vi "Fault Handling.vi"(8 "error in (no error)":errorcluster, 10 "FaultCode":i32, 11 "OPC UA in":refnum<class "OPC UA.lvclass">) -> (0 "error out":errorcluster, 2 "Fault codes":cluster{"Bit":string, "Description":string}[](array[cluster]), 3 "OPC UA out":refnum<class "OPC UA.lvclass">)   [LabVIEW 2021, in "OPC UA.lvlib" / "OPC UA.lvclass"]
uses:
  OPC UA.lvclass
  OPC UA.lvclass/OPC UA.ctl
panel:
  out "Fault":bool
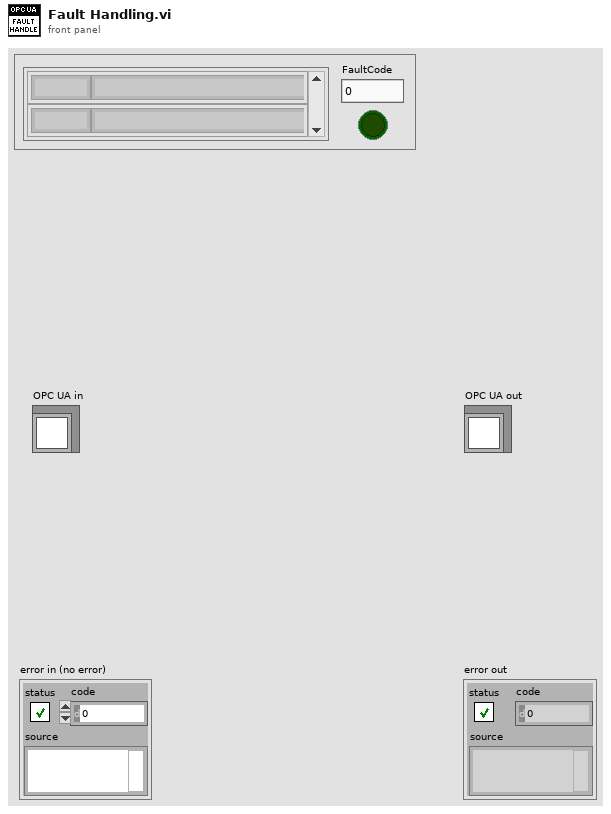
[diagram p1: front panel]
types:
  T1 = enum32{"Invalid", "Standard", "Closed", "Hidden", "Minimized", "Maximized"}
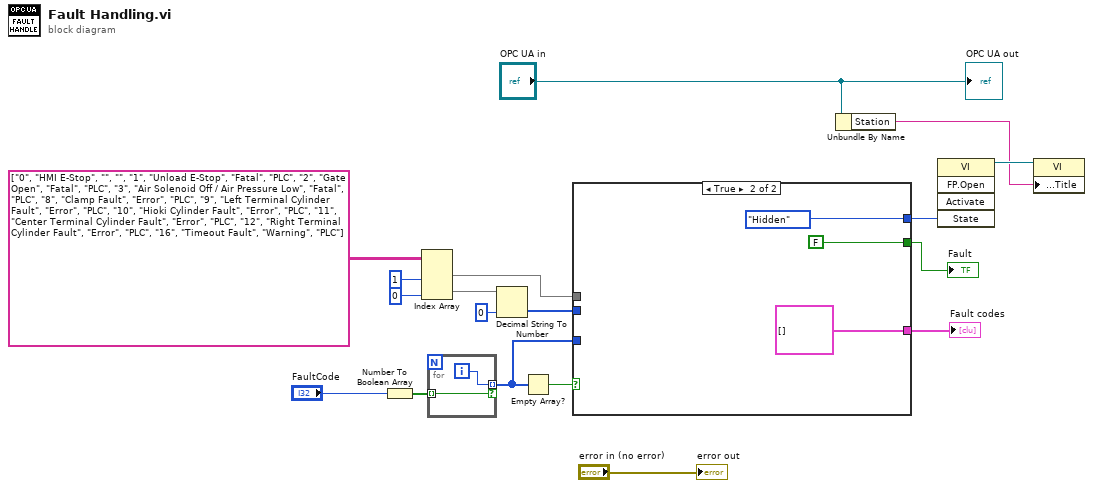
[diagram p0: block diagram]
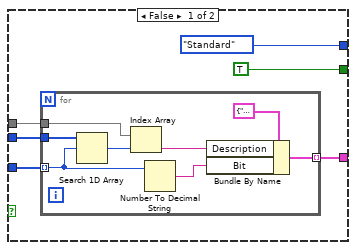
[diagram p2: hidden frame]
diagram:
  n1 = Number To Boolean Array(number="FaultCode") -> (Boolean array=w11:bool[])
  n2 = Index Array(array=string[][] [["0", "HMI E-Stop", "", ""], ["1", "Unload E-Stop", "Fatal", "PLC"], ["2", "Gate Open", "Fatal", "PLC"], ["3", "Air Solenoid Off / Air Pressure Low", "Fatal", "PLC"], ["8", "Clamp Fault", "Error", "PLC"], ["9", "Left Terminal Cylinder Fault", "Error", "PLC"], ["10", "Hioki Cylinder Fault", "Error", "PLC"], ["11", "Center Terminal Cylinder Fault", "Error", "PLC"], ["12", "Right Terminal Cylinder Fault", "Error", "PLC"], ["16", "Timeout Fault", "Warning", "PLC"]], index (col) #1=1 ("disabled index (col)"), index (col) #2=0 ("index (col)")) -> (element #1=w5:string[], element #2=w13:string[])  [unwired: 2 in]
  n3 = for {
    tunnel: w11 -> [w19] mode=indexing
    tunnel: [w20] -> w8 mode=indexing if=w19
    i -> [w20]
  }
  n4 = Decimal String To Number(string=w13, default (0L)=0 ("default (0 I32)")) -> (number=w7:i32[])  [unwired: 1 in, 1 out]
  n5 = Empty Array?(array=w8) -> (empty?=w6:bool)
  n6 = case shown="True" w6 {
    tunnel: [T1."Standard" ("State") T1."Hidden" ("State")] -> w14
    tunnel: [w21 cluster{"Bit":string, "Description":string}[] []] -> w2
    tunnel: [TRUE FALSE] -> w1
    tunnel: w7 -> [w24 _]
    tunnel: w8 -> [w23 _]
    tunnel: w5 -> [w22 _]
    frame False {
      n7 = for {
        tunnel: w23 -> [w29] mode=indexing
        tunnel: w24 -> [w34]
        tunnel: w22 -> [w32]
        tunnel: [w28] -> w21 mode=indexing
        n8 = Search 1D Array(1D array=w34, element=w29) -> (index of element=w33:i32)  [unwired: 1 in]
        n9 = Index Array(array=w32, index=w33) -> (element=w30:string)
        n10 = Number To Decimal String(number=w29) -> (decimal integer string=w27:string)  [unwired: 1 in]
        n11 = Bundle By Name(cluster=cluster{"Bit":string, "Description":string} {"Bit"="", "Description"=""} ("Fault"), "Description"=w30, "Bit"=w27) -> (w28:cluster{"Bit":string, "Description":string})
      }
    }
    frame True {
    }
  }
  "Fault" <- w1
  "Fault codes" <- w2
  n12 = Unbundle By Name("OPC UA in") -> ("Station"=w16:string)
  n13 = invoke class="VI" method="FP.Open"("State"=w14) -> (reference out=w18:refnum<vi>)  [unwired: 4 in, 4 out]
  n14 = property class="VI"(reference=w18, "Front Panel.Title"=w16) -> ()  [unwired: 1 in, 2 out]
  "error out" <- "error in (no error)"
  "OPC UA out" <- "OPC UA in"
